vi "PreviewSnapshot.vi"(8 "Error In":errorcluster, 10 "Preview?":bool=TRUE, 11 "SystemSnapshot":T1) -> (0 "Error Out":errorcluster, 2 "Install Command":string, 3 "Preview":string)   [LabVIEW 2019, in "CEPM.lvlib"]
uses:
  CEPM.lvlib
  Typedefs/SystemSnapshot.ctl
  <vilib>/National Instruments/NIPM API (Beta)/NIPM_API.lvlib
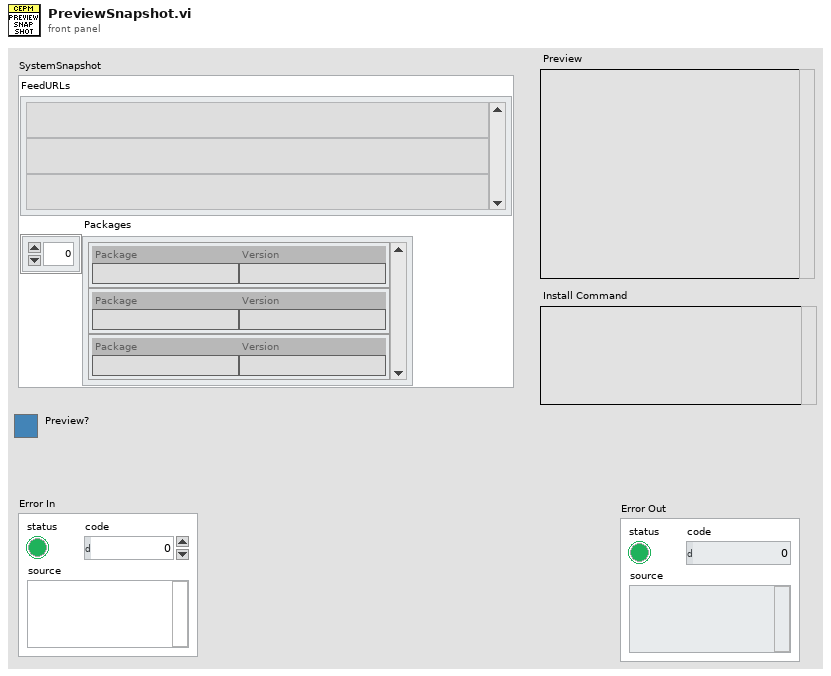
[diagram p1: front panel]
types:
  T1 = typedef "CEPM.lvlib/SystemSnapshot.ctl" = cluster{"FeedURLs":string[], "Packages":cluster{"Package":string, "Version":string}[]}
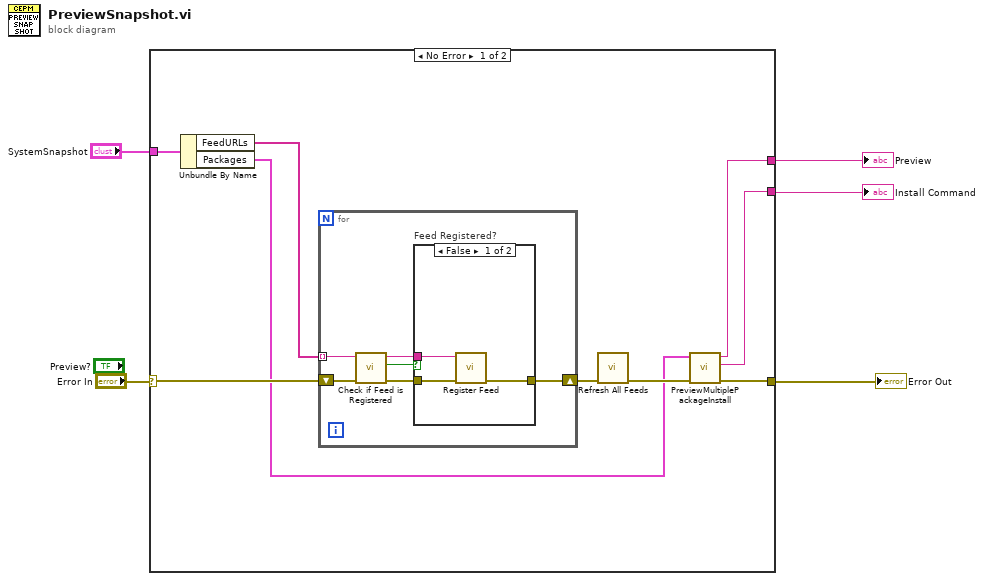
[diagram p0: block diagram]
diagram:
  n1 = case shown="No Error" "Error In" {
    selector: "Error In" -> [w11 w25]
    tunnel: [w9 w25] -> w4
    tunnel: "SystemSnapshot" -> [w14 _]
    tunnel: [w7 _] -> w2
    tunnel: [w6 _] -> w1
    frame No Error {
      n2 = Unbundle By Name(w14) -> ("FeedURLs"=w12:string[], "Packages"=w8:cluster{"Package":string, "Version":string}[])
      n3 = for {
        shift-right: [w20] -> w13
        shift-left: w11 -> [w19]
        tunnel: w12 -> [w17] mode=indexing
        n4 = call <vilib>:"Check if Feed is Registered.vi"("error in"=w19, "feed URI"=w17) -> ("error out"=w18:errorcluster, "feed URI registered?"=w15:bool, "feed URI out"=w16:string)  [unwired: 6 in, 1 out]
        n5 = case "Feed Registered?" shown="False" w15 {
          tunnel: [w23 w24] -> w20
          tunnel: w18 -> [w22 w24]
          tunnel: w16 -> [w21 _]
          frame False {
            n6 = call <vilib>:"Register Feed.vi"("error in"=w22, "feed URI"=w21) -> ("error out"=w23:errorcluster)  [unwired: 8 in, 1 out]
          }
          frame True {
          }
        }
      }
      n7 = call <vilib>:"Refresh All Feeds.vi"("error in"=w13) -> ("error out"=w10:errorcluster)  [unwired: 9 in, 1 out]
      n8 = call "PreviewMultiplePackageInstall.vi"("Error In"=w10, "Packages"=w8) -> ("Error Out"=w9:errorcluster, "Install Command"=w6:string, "Preview"=w7:string)  [unwired: 7 in]
    }
    frame Error {
    }
  }
  "Error Out" <- w4
  "Preview" <- w2
  "Install Command" <- w1
